vi "PPMS.Set Temperature.vi"(8 "error in (no error)":errorcluster, 10 "Data":variant, 11 "instrument.PPMS":refnum<class "instrument.PPMS.lvclass">) -> (0 "error out":errorcluster, 3 "instrument.PPMS out":refnum<class "instrument.PPMS.lvclass">)   [LabVIEW 2019, in "instrument.PPMS.lvclass"]
uses:
  instrument.PPMS.lvclass
  instrument.PPMS.lvclass/instrument.PPMS.ctl
  <userlib>/LevyLab/Levylab Instruments/Instrument Types/Cryostat/Typedefs/Set Temperature--cluster.ctl
  <userlib>/LevyLab/Levylab Instruments/Instrument Types/Cryostat/Instrument.Cryostat.lvclass
  38aab25a-2199-4090-9f7e-cb0166537263.vi
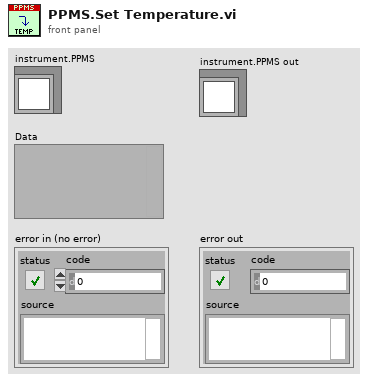
[diagram p1: front panel]
types:
  T1 = typedef "Instrument.Cryostat.lvclass/Set Temperature--cluster.ctl" = cluster{"Temperature (K)":dbl, "Rate (K/min)":dbl, "Channel":i32}
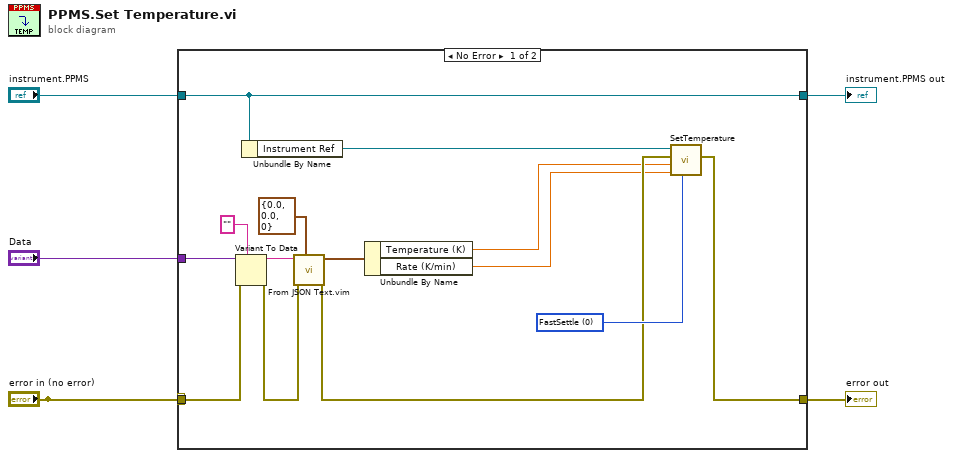
[diagram p0: block diagram]
diagram:
  n1 = case shown="No Error" "error in (no error)" {
    selector: "error in (no error)" -> [_ w21]
    tunnel: "Data" -> [w13 _]
    tunnel: [w18 w21] -> w4
    tunnel: "instrument.PPMS" -> [w16 w20]
    tunnel: [w16 w20] -> w2
    tunnel: "error in (no error)" -> [w12 _]
    frame No Error {
      w19 = 0 items=["FastSettle", "NoOvershoot"] ("Approach")
      n2 = Variant To Data(error in=w12, type="", Variant=w13) -> (data=w10:string, error out=w11:errorcluster)
      n3 = Unbundle By Name(w16) -> ("Instrument Ref"=w17:refnum<k24>)
      n4 = call "From JSON Text.vim"("Data Type and Default Value"=T1 {"Temperature (K)"=0.0, "Rate (K/min)"=0.0, "Channel"=0} ("Set Temperature"), "error in (no error)"=w11, "JSON"=w10) -> ("error out"=w9:errorcluster, "Data out"=w8:T1)  [unwired: 7 in]
      n5 = Unbundle By Name(w8) -> ("Temperature (K)"=w7:dbl, "Rate (K/min)"=w6:dbl)
      n6 = call "SetTemperature.vi"("Approach"=w19, "Rate"=w6, "Temperature"=w7, "error in (no error)"=w9, "Instrument Ref In"=w17) -> ("error out"=w18:errorcluster)  [unwired: 2 in, 2 out]
    }
    frame Error {
    }
  }
  "error out" <- w4
  "instrument.PPMS out" <- w2
